vi "test-swerve-drive-kinematics-14.vi"() -> (3 "Test Passed":bool)   [LabVIEW 2019]
uses:
  <vilib>/Rock Robotics/WPI/ThirdParty/JAS_Junk/TrajLib/Conv_Deg_Radians.vi
  <vilib>/Rock Robotics/WPI/ThirdParty/JAS_Junk/TrajLib/Rotation2d_CreateAngle.vi
  <vilib>/Rock Robotics/WPI/ThirdParty/JAS_Junk/TrajLib/Trajectory_Library.lvlib
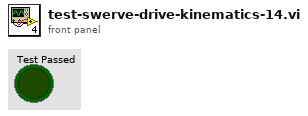
[diagram p1: front panel]
types:
  T1 = typedef "Trajectory_Library.lvlib/TRANSLATION2D.ctl" = cluster{"X":dbl, "Y":dbl}
  T2 = typedef "Trajectory_Library.lvlib/ROTATION2D.ctl" = cluster{"VALUE":dbl, "COS":dbl, "SIN":dbl}
  T3 = typedef "Trajectory_Library.lvlib/SWERVE_DRIVE_MODULE_POSITION.ctl" = cluster{"Distance":dbl, "Angle":T2}
  T4 = typedef "Trajectory_Library.lvlib/SWERVE_DRIVE_KINEMATICS.ctl" = cluster{"NumModules":i32, "InverseKinematics":T5, "ForwardKinematics":T5, "Modules":T1[], "PrevCoR":T1, "SavedModuleStates":T6[]}
  T5 = typedef "NI_Matrix.lvlib/RealMatrix.ctl" = dbl[][]
  T6 = typedef "Trajectory_Library.lvlib/SWERVE_DRIVE_MODULE_STATE.ctl" = cluster{"Speed":dbl, "Angle":T2}
  T7 = typedef "Trajectory_Library.lvlib/TWIST2D.ctl" = cluster{"dX":dbl, "dY":dbl, "dTHETA":dbl}
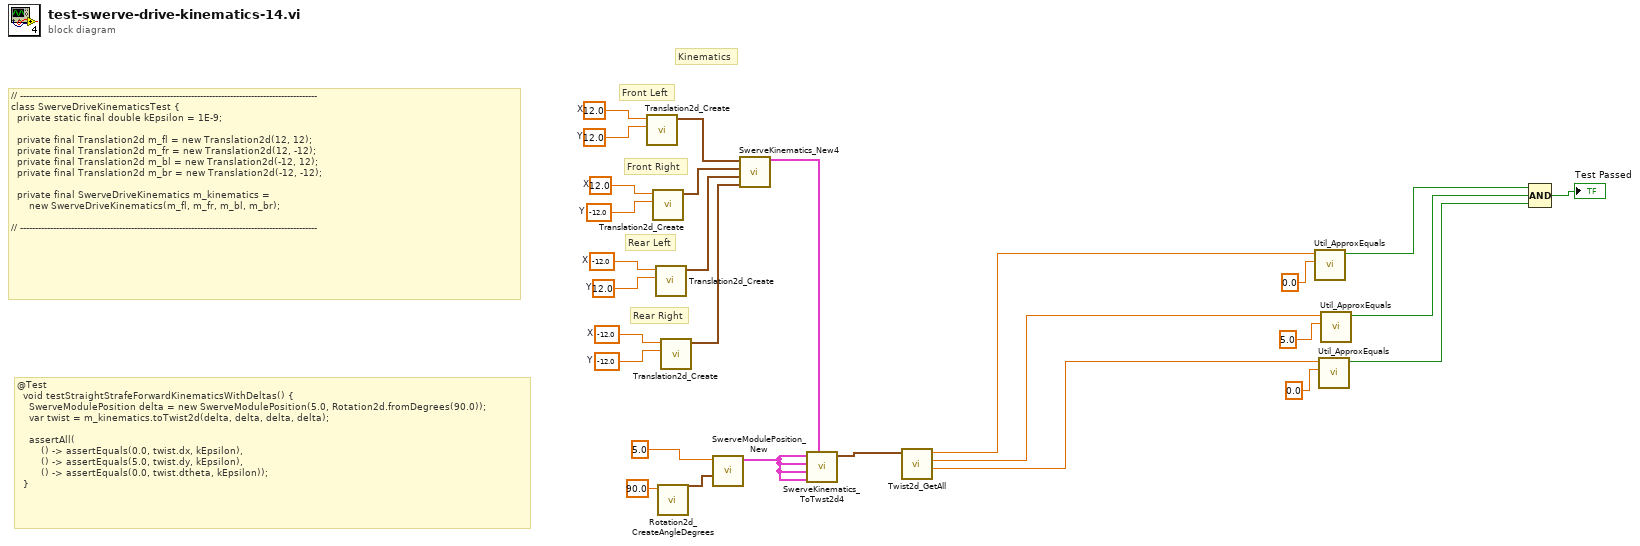
[diagram p0: block diagram]
diagram:
  w24 = -12.0  # X
  w23 = -12.0  # Y
  w22 = -12.0  # X
  w21 = 12.0  # Y
  w20 = 12.0  # X
  w19 = -12.0  # Y
  w18 = 12.0  # X
  w17 = 12.0  # Y
  # "@Test\n  void testStraightStrafeForwardKinematicsWithDeltas() {\n    SwerveModulePosition delta = new SwerveModulePosition(5.0, Rotation2d.fromDegrees(90.0));\n    var twist = m_kinematics.toTwist2d(delta, delta, delta, delta);\n\n    assertAll(\n        () -> assertEquals(0.0, twist.dx, kEpsilon),\n        () -> assertEquals(5.0, twist.dy, kEpsilon),\n        () -> assertEquals(0.0, twist.dtheta, kEpsilon));\n  }"
  # "Kinematics"
  # "Rear Right"
  # "Rear Left"
  # "Front Right"
  # "Front Left"
  # "// ---------------------------------------------------------------------------------------------------\nclass SwerveDriveKinematicsTest {\n  private static final double kEpsilon = 1E-9;\n\n  private final Translation2d m_fl = new Translation2d(12, 12);\n  private final Translation2d m_fr = new Translation2d(12, -12);\n  private final Translation2d m_bl = new Translation2d(-12, 12);\n  private final Translation2d m_br = new Translation2d(-12, -12);\n\n  private final SwerveDriveKinematics m_kinematics =\n      new SwerveDriveKinematics(m_fl, m_fr, m_bl, m_br);\n\n// ---------------------------------------------------------------------------------------------------"
  n1 = call <vilib>:"Translation2d_Create.vi"("Y"=w17, "X"=w18) -> ("TRANSLATION"=w25:T1)  [unwired: 9 in]
  n2 = call <vilib>:"Translation2d_Create.vi"("Y"=w19, "X"=w20) -> ("TRANSLATION"=w26:T1)  [unwired: 9 in]
  n3 = call <vilib>:"Translation2d_Create.vi"("Y"=w21, "X"=w22) -> ("TRANSLATION"=w27:T1)  [unwired: 9 in]
  n4 = call <vilib>:"Rotation2d_CreateAngleDegrees.vi"("Angle_Degrees"=90.0) -> ("ROTATION"=w9:T2)  [unwired: 10 in]
  n5 = call <vilib>:"Translation2d_Create.vi"("Y"=w23, "X"=w24) -> ("TRANSLATION"=w28:T1)  [unwired: 9 in]
  n6 = call <vilib>:"SwerveModulePosition_New.vi"("ROTATION"=w9, "Distance"=5.0 ("Speed")) -> ("SWERVE_DRIVE_MODULE_POSITION"=w5:T3)  [unwired: 9 in]
  n7 = call <vilib>:"SwerveKinematics_New4.vi"("wheel 3"=w28, "wheel 2"=w27, "wheel 1"=w26, "wheel 0"=w25) -> ("SWERVE_DRIVE_KINEMATICS"=w6:T4)  [unwired: 7 in]
  n8 = call <vilib>:"SwerveKinematics_ToTwst2d4.vi"("in SWERVE_DRIVE_KINEMATICS"=w6, "Wheel Delta 3"=w5, "Wheel Delta 2"=w5, "Wheel Delta 1"=w5, "Wheel Delta 0"=w5) -> ("Twist2d"=w4:T7)  [unwired: 5 in, 1 out]
  n9 = call <vilib>:"Twist2d_GetAll.vi"("TWIST"=w4) -> ("dTHETA"=w1:dbl, "dY"=w2:dbl, "dX"=w3:dbl)  [unwired: 8 in]
  n10 = call <vilib>:"Util_ApproxEquals.vi"("Value 2"=0.0, "Value 1"=w3) -> ("ApproxEquals"=w13:bool)  [unwired: 9 in]
  n11 = call <vilib>:"Util_ApproxEquals.vi"("Value 2"=0.0, "Value 1"=w1) -> ("ApproxEquals"=w11:bool)  [unwired: 9 in]
  n12 = call <vilib>:"Util_ApproxEquals.vi"("Value 2"=5.0, "Value 1"=w2) -> ("ApproxEquals"=w12:bool)  [unwired: 9 in]
  n13 = Compound Arithmetic op=AND(w13, w12, w11) -> (→"Test Passed":bool)
